vi "test_CalculateSpecificationBuildOrder_SampleProject.vi"() -> (3 "Pass?":bool)   [LabVIEW 2019, in "Tests.SolutionBuilder.lvlib"]
uses:
  Tests.SolutionBuilder.lvlib
  SolutionBuilder/SolutionBuilder.lvclass
  SolutionBuilder/ProjectItem/ProjectItem.lvclass
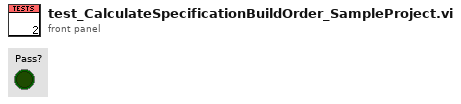
[diagram p1: front panel]
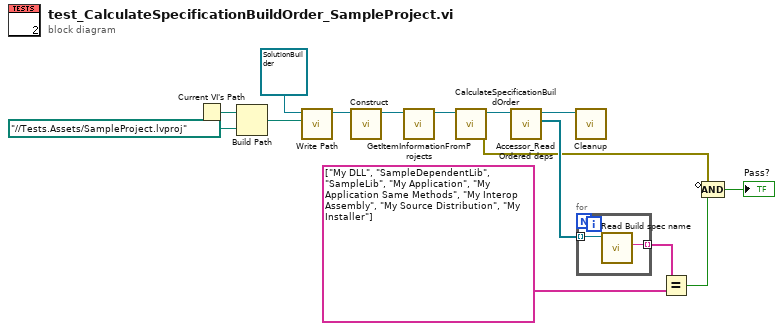
[diagram p0: block diagram]
diagram:
  n1 = Current VI's Path() -> (path=w14:path)
  n2 = Build Path(base path=w14, name or relative path=path "../../Tests.Assets/SampleProject.lvproj" ("Path")) -> (appended path=w12:path)
  n3 = call "Write Path.vi"("Path"=w12, "SolutionBuilder in"=refnum<class "SolutionBuilder.lvclass"> refnum) -> ("SolutionBuilder out"=w11:refnum<class "SolutionBuilder.lvclass">)  [unwired: 9 in]
  n4 = call "Construct.vi"("SolutionBuilder in"=w11) -> ("SolutionBuilder out"=w9:refnum<class "SolutionBuilder.lvclass">)  [unwired: 9 in, 1 out]
  n5 = call "GetItemInformationFromProjects.vi"("SolutionBuilder in"=w9) -> ("SolutionBuilder out"=w8:refnum<class "SolutionBuilder.lvclass">)  [unwired: 9 in, 1 out]
  n6 = call "CalculateSpecificationBuildOrder.vi"("SolutionBuilder in"=w8) -> ("error out"=w4:errorcluster, "SolutionBuilder out"=w7:refnum<class "SolutionBuilder.lvclass">)  [unwired: 9 in]
  n7 = call "Accessor_Read Ordered deps.vi"("SolutionBuilder in"=w7) -> ("Ordered deps"=w5:refnum<class "ProjectItem.lvclass">[], "SolutionBuilder out"=w6:refnum<class "SolutionBuilder.lvclass">)  [unwired: 8 in, 1 out]
  n8 = call "Cleanup.vi"("SolutionBuilder in"=w6) -> ()  [unwired: 9 in, 2 out]
  n9 = for {
    tunnel: w5 -> [w17] mode=indexing
    tunnel: [w16] -> w3 mode=indexing
    n10 = call "Read Build spec name.vi"("ProjectItem in"=w17) -> ("Build spec name"=w16:string)  [unwired: 9 in, 1 out]
  }
  n11 = Equal?(x=w3, y=string[] ["My DLL", "SampleDependentLib", "SampleLib", "My Application", "My Application Same Methods", "My Interop Assembly", "My Source Distribution", "My Installer"] ("Array")) -> (x = y?=w10:bool)
  n12 = Compound Arithmetic op=AND(invert w4, w10) -> (→"Pass?":bool)
